vi "lockin_host.vi"() -> ()   [LabVIEW 2009]
uses:
  <vilib>/rvi/interface/nirviOpenFPGA/nirviOpenFPGA.xnode
  FPGA Bitfiles/fpga_lockin.lvproj_FPGA Target_lockin_fpga.vi.lvbitx
  lockin_fpga.vi
  <vilib>/FPGAPlugInAG/Pxi-7841r/nirviIntfOpen_PXI-7841R.vi
  <vilib>/rvi/interface/nirviMethod/nirviMethod.xnode
  <vilib>/Utility/error.llb/Merge Errors.vi
  <vilib>/LabVIEW Targets/FPGA/Rio/nirio_HostInterface/nirio_DMAStopAll.vi
  <vilib>/rvi/interface/common/niFpgaNodeNameForErrorReporting.ctl
  <vilib>/rvi/errors/niLvFpgaWhatHappensToTopLevelVI.ctl
  <vilib>/LabVIEW Targets/FPGA/Rio/nirio_HostInterface/nirio_DisableInterrupts.vi
  <vilib>/Utility/error.llb/Error Cluster From Error Code.vi
  <vilib>/rvi/errors/niLvFpgaAdjustHostInterfaceError.vi
  <vilib>/LabVIEW Targets/FPGA/Rio/nirio_HostInterface/nirio_Reset.vi
  <vilib>/RVI Host/nirviSupport.llb/nirviErrorClusterFromErrorCode.vi
  <vilib>/LabVIEW Targets/FPGA/Rio/nirio_HostInterface/nirio_EnableInterrupts.vi
  <vilib>/rvi/errors/niLvFpgaReportInternalErrorWithAdditionalInfo.vi
  <vilib>/rvi/interface/nirviReadWriteControl/nirviReadWriteControl.xnode
  <vilib>/rvi/interface/nirviCloseFPGA/nirviCloseFPGA.xnode
  <vilib>/FPGAPlugInAG/Pxi-7841r/nirviIntfClose_PXI-7841R.vi
  <vilib>/userDefined/High Color/nirio_resource_hc.ctl
  NiRioSrv.dll
panel:
  in  "Time Constant [s] 4":dbl caption="Time Constant [s]"
  out "Y [V] 4":dbl caption="Y [V]"
  out "Phase [Deg] 4":dbl caption="Phase [Deg]"
  out "R [V] 4":dbl caption="R [V]"
  out "X [V] 4":dbl
  out "Filter Rolloff 4":enum8{"6 dB", "12 dB", "18 dB", "24 dB"}(ring) caption="Filter Rolloff"
  in  "Amplitude [V] 4":dbl caption="Amplitude [V]"
  in  "Frequency [Hz] 4":dbl caption="Frequency [Hz]"
  in  "Phase [Deg] 4":dbl caption="Phase [Deg]"
  in  "Time Constant [s] 3":dbl caption="Time Constant [s]"
  out "Y [V] 3":dbl caption="Y [V]"
  out "Phase [Deg] 3":dbl caption="Phase [Deg]"
  out "R [V] 3":dbl caption="R [V]"
  out "X [V] 3":dbl
  out "Filter Rolloff 3":enum8{"6 dB", "12 dB", "18 dB", "24 dB"}(ring) caption="Filter Rolloff"
  in  "Amplitude [V] 3":dbl caption="Amplitude [V]"
  in  "Frequency [Hz] 3":dbl caption="Frequency [Hz]"
  in  "Phase [Deg] 3":dbl caption="Phase [Deg]"
  in  "Time Constant [s] 2":dbl caption="Time Constant [s]"
  out "Y [V] 2":dbl caption="Y [V]"
  out "Phase [Deg] 2":dbl caption="Phase [Deg]"
  out "R [V] 2":dbl caption="R [V]"
  out "X [V] 2":dbl
  out "Filter Rolloff 2":enum8{"6 dB", "12 dB", "18 dB", "24 dB"}(ring) caption="Filter Rolloff"
  in  "Amplitude [V] 2":dbl caption="Amplitude [V]"
  in  "Frequency [Hz] 2":dbl caption="Frequency [Hz]"
  in  "Phase [Deg] 2":dbl caption="Phase [Deg]"
  in  "Time Constant [s] 1":dbl caption="Time Constant [s]"
  out "Y [V] 1":dbl caption="Y [V]"
  out "Phase [Deg] 1":dbl caption="Phase [Deg]"
  out "R [V] 1":dbl caption="R [V]"
  out "X [V] 1":dbl
  in  "Data Rate [Hz]":dbl
  out "Filter Rolloff 1":enum8{"6 dB", "12 dB", "18 dB", "24 dB"}(ring) caption="Filter Rolloff"
  in  "stop":bool
  in  "Update Freq [Hz]":dbl
  in  "Amplitude [V] 1":dbl caption="Amplitude [V]"
  in  "Frequency [Hz] 1":dbl caption="Frequency [Hz]"
  in  "Phase [Deg] 1":dbl caption="Phase [Deg]"
  # "Lockin Amplifier 1"
  # "Lockin Amplifier 3"
  # "Filter Settings"
  # "Output"
  # "Filter Settings"
  # "Output"
  # "Reference Signal Settings"
  # "Reference Signal Settings"
  # "Lockin Amplifier 2"
  # "Lockin Amplifier 4"
  # "Filter Settings"
  # "Output"
  # "Filter Settings"
  # "Output"
  # "Global"
  # "Reference Signal Settings"
  # "Reference Signal Settings"
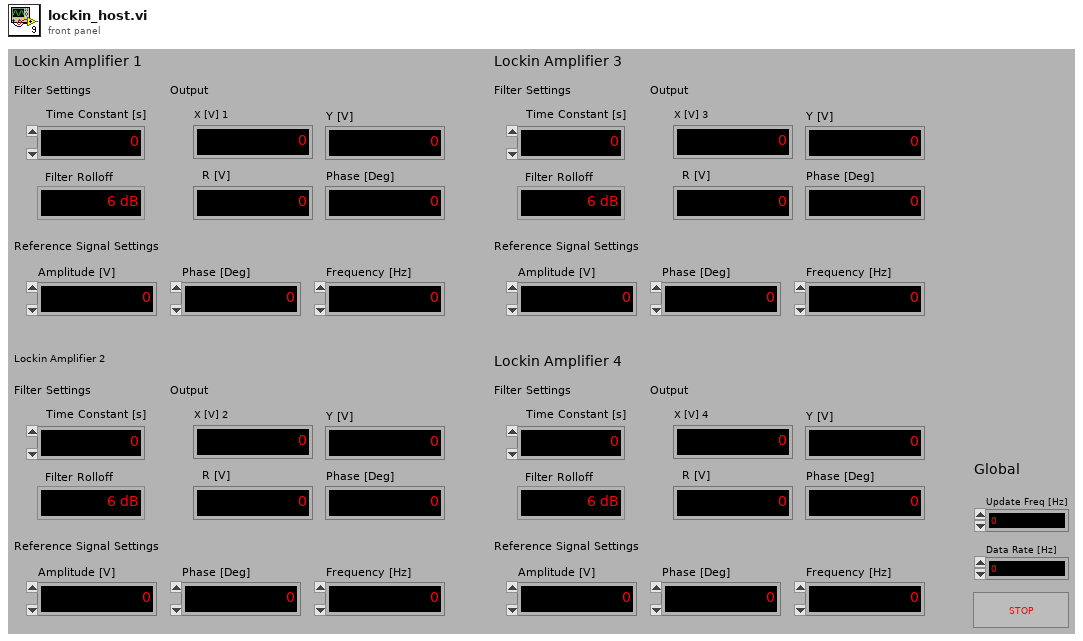
[diagram p1: front panel]
types:
  T1 = typedef "niFpgaNodeNameForErrorReporting.ctl" = enum16{"Open FPGA VI Reference", "Read/Write Control", "Invoke Method: Abort", "Invoke Method: Acknowledge IRQ", "Invoke Method: Download", "Invoke Method: FIFO.Configure", "Invoke Method: FIFO.Read", "Invoke Method: FIFO.Start", "Invoke Method: FIFO.Stop", "Invoke Method: FIFO.Write", "Invoke Method: Reset", "Invoke Method: Run", "Invoke Method: Wait on IRQ", "Close FPGA VI Reference"}
  T2 = typedef "niLvFpgaWhatHappensToTopLevelVI.ctl" = enum16{"top level VI scripted behind XNode", "top level VI inlined behind XNode"}
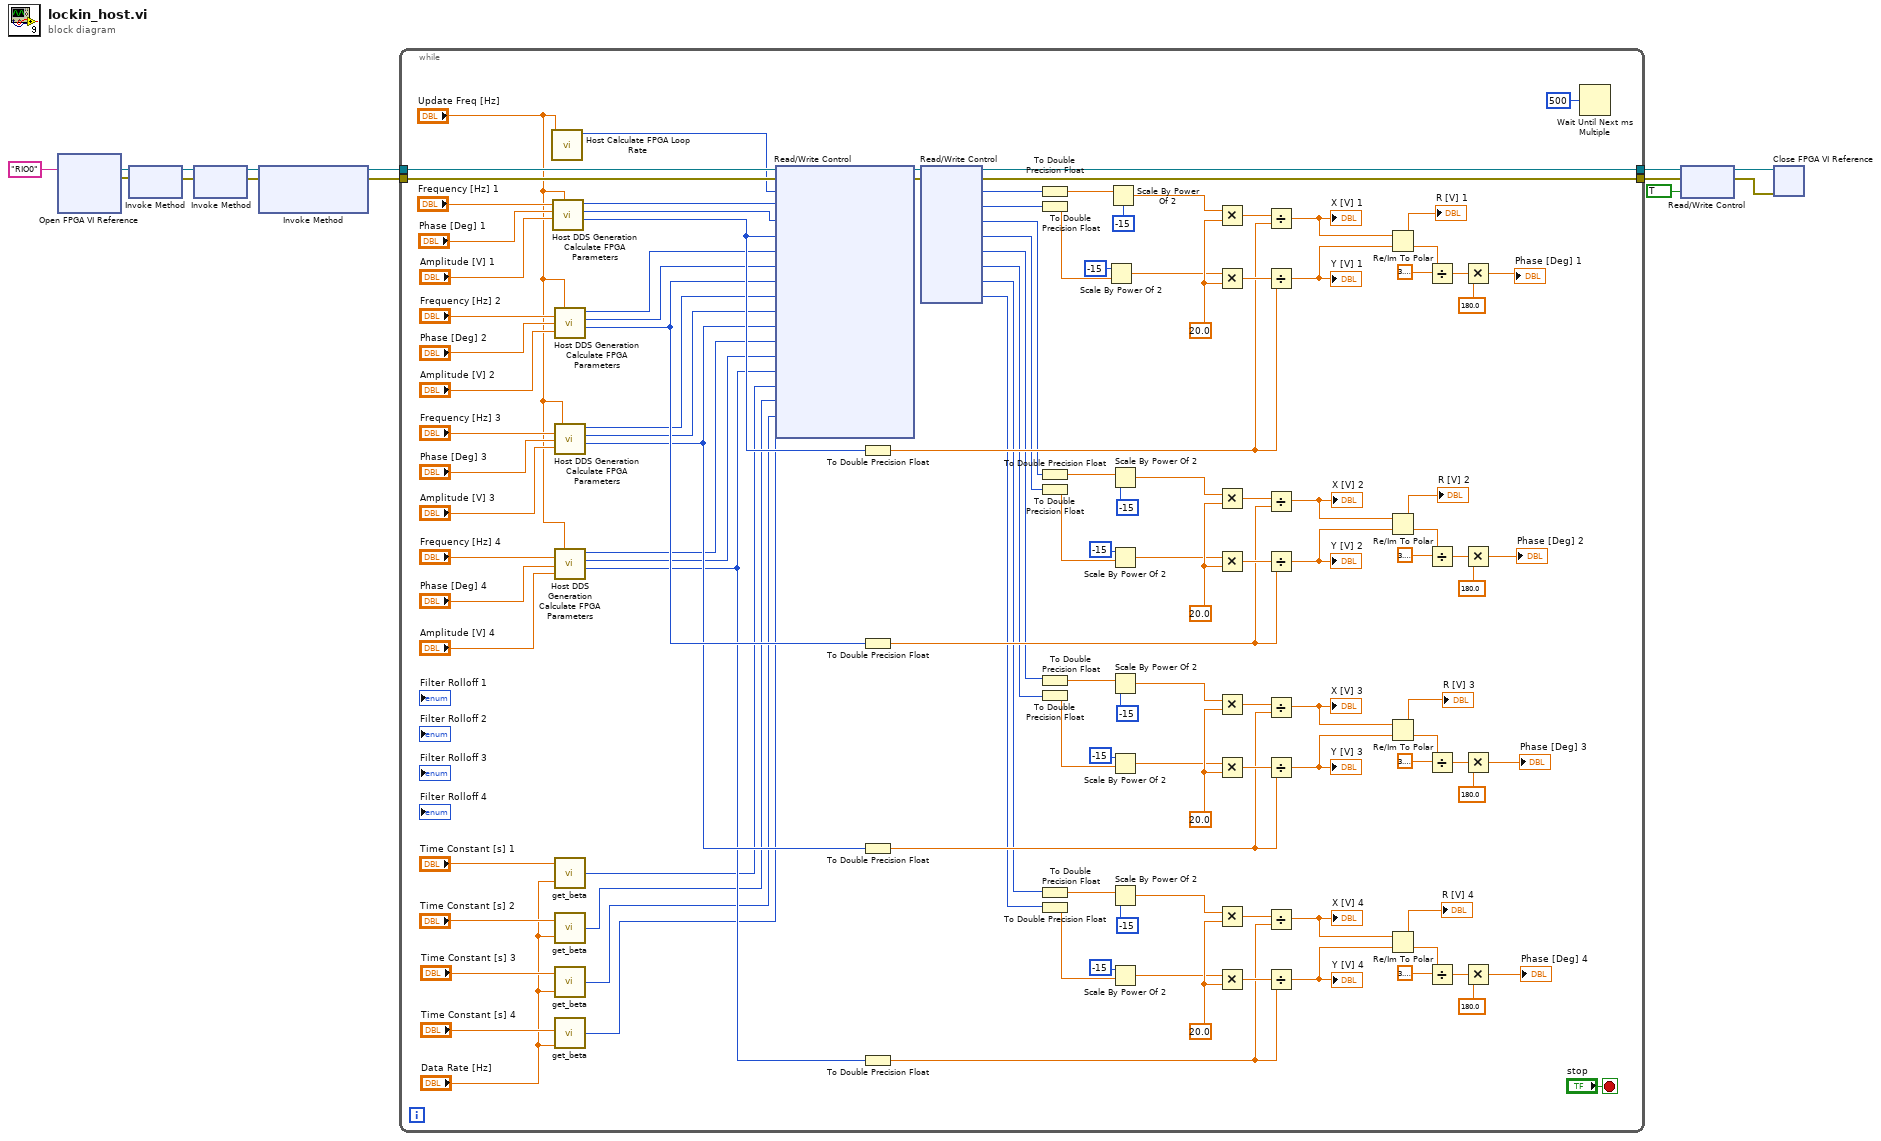
[diagram p0: block diagram]
diagram:
  n1 = xnode "Open FPGA VI Reference"("resource name"="RIO0") -> ("FPGA VI Reference Out"=w9:refnum<k20>, "error out"=w8:errorcluster)  [unwired: 1 in]
  n2 = xnode "Invoke Method"("FPGA VI Reference In"=w9, "error in"=w8) -> ("FPGA VI Reference Out"=w13:refnum<k20>, "error out"=w12:errorcluster)
  n3 = xnode "Invoke Method"("FPGA VI Reference In"=w13, "error in"=w12) -> ("FPGA VI Reference Out"=w11:refnum<k20>, "error out"=w10:errorcluster)
  n4 = xnode "Invoke Method"("FPGA VI Reference In"=w11, "error in"=w10) -> ("FPGA VI Reference Out"=w7:refnum<k20>, "error out"=w6:errorcluster)  [unwired: 1 out]
  n5 = while {
    tunnel: w7 -> [w133]
    tunnel: w6 -> [w132]
    tunnel: [w126] -> w3
    tunnel: [w125] -> w2
    stop <- "stop" stop-if-true
    w44 = 20.0
    w83 = 20.0
    w108 = 20.0
    w100 = 20.0
    n6 = call "Host Calculate FPGA Loop Rate.vi"("Loop Frequency (Hz)"="Update Freq [Hz]") -> ("Loop  Rate (ticks)"=w131:u32)  [unwired: 10 in]
    n7 = call "Host DDS Generation Calculate FPGA Parameters.vi"("Loop Rate (Hz)"="Update Freq [Hz]", "Signal Amplitude (V)"="Amplitude [V] 1", "Phase Shift (Deg)"="Phase [Deg] 1", "DDS Signal Frequency (Hz)"="Frequency [Hz] 1") -> ("AO Amplitude"=w119:u16, "Phase Shift Sin"=w129:u32, "Accumulator Increment"=w130:u32)  [unwired: 3 in, 2 out]
    n8 = call "Host DDS Generation Calculate FPGA Parameters.vi"("Loop Rate (Hz)"="Update Freq [Hz]", "Signal Amplitude (V)"="Amplitude [V] 2", "Phase Shift (Deg)"="Phase [Deg] 2", "DDS Signal Frequency (Hz)"="Frequency [Hz] 2") -> ("AO Amplitude"=w103:u16, "Phase Shift Sin"=w111:u32, "Accumulator Increment"=w112:u32)  [unwired: 3 in, 2 out]
    n9 = call "Host DDS Generation Calculate FPGA Parameters.vi"("Loop Rate (Hz)"="Update Freq [Hz]", "Signal Amplitude (V)"="Amplitude [V] 3", "Phase Shift (Deg)"="Phase [Deg] 3", "DDS Signal Frequency (Hz)"="Frequency [Hz] 3") -> ("AO Amplitude"=w72:u16, "Phase Shift Sin"=w86:u32, "Accumulator Increment"=w87:u32)  [unwired: 3 in, 2 out]
    n10 = call "Host DDS Generation Calculate FPGA Parameters.vi"("Loop Rate (Hz)"="Update Freq [Hz]", "Signal Amplitude (V)"="Amplitude [V] 4", "Phase Shift (Deg)"="Phase [Deg] 4", "DDS Signal Frequency (Hz)"="Frequency [Hz] 4") -> ("AO Amplitude"=w32:u16, "Phase Shift Sin"=w47:u32, "Accumulator Increment"=w48:u32)  [unwired: 3 in, 2 out]
    n11 = call "get_beta.vi"("Data Rate [Hz]"="Data Rate [Hz]", "Time Constant [s]"="Time Constant [s] 1") -> ("beta"=w16:i32)
    n12 = call "get_beta.vi"("Data Rate [Hz]"="Data Rate [Hz]", "Time Constant [s]"="Time Constant [s] 2") -> ("beta"=w17:i32)
    n13 = call "get_beta.vi"("Data Rate [Hz]"="Data Rate [Hz]", "Time Constant [s]"="Time Constant [s] 3") -> ("beta"=w18:i32)
    n14 = call "get_beta.vi"("Data Rate [Hz]"="Data Rate [Hz]", "Time Constant [s]"="Time Constant [s] 4") -> ("beta"=w19:i32)
    n15 = xnode "Read/Write Control"("FPGA VI Reference In"=w133, "error in"=w132, "Update Rate (ticks)"=w131, "Accumulator Increment 1"=w130, "Phase Shift 1"=w129, "Signal Amplitude 1"=w119, "Accumulator Increment 2"=w112, "Phase Shift 2"=w111, "Signal Amplitude 2"=w103, "Accumulator Increment 3"=w87, "Phase Shift 3"=w86, "Signal Amplitude 3"=w72, "Accumulator Increment 4"=w48, "Phase Shift 4"=w47, "Signal Amplitude 4"=w32, "beta1"=w16, "beta2"=w17, "beta3"=w18, "beta4"=w19) -> ("FPGA VI Reference Out"=w128:refnum<k20>, "error out"=w127:errorcluster)
    n16 = To Double Precision Float(number=w119) -> (double precision float=w118:dbl)
    n17 = To Double Precision Float(number=w103) -> (double precision float=w102:dbl)
    n18 = To Double Precision Float(number=w72) -> (double precision float=w71:dbl)
    n19 = To Double Precision Float(number=w32) -> (double precision float=w33:dbl)
    n20 = xnode "Read/Write Control"("FPGA VI Reference In"=w128, "error in"=w127) -> ("FPGA VI Reference Out"=w126:refnum<k20>, "error out"=w125:errorcluster, "X_fpga 1"=w27:i32, "Y_fpga 1"=w26:i32, "X_fpga 2"=w25:i32, "Y_fpga 2"=w24:i32, "X_fpga 3"=w23:i32, "Y_fpga 3"=w22:i32, "X_fpga 4"=w21:i32, "Y_fpga 4"=w20:i32)
    n21 = To Double Precision Float(number=w27) -> (double precision float=w96:dbl)
    n22 = To Double Precision Float(number=w26) -> (double precision float=w98:dbl)
    n23 = To Double Precision Float(number=w25) -> (double precision float=w93:dbl)
    n24 = To Double Precision Float(number=w24) -> (double precision float=w90:dbl)
    n25 = To Double Precision Float(number=w23) -> (double precision float=w78:dbl)
    n26 = To Double Precision Float(number=w22) -> (double precision float=w75:dbl)
    n27 = To Double Precision Float(number=w21) -> (double precision float=w39:dbl)
    n28 = To Double Precision Float(number=w20) -> (double precision float=w36:dbl)
    n29 = Scale By Power Of 2(n=-15, x=w98) -> (x*2^n=w99:dbl)
    n30 = Scale By Power Of 2(n=-15, x=w96) -> (x*2^n=w94:dbl)
    n31 = Scale By Power Of 2(n=-15, x=w93) -> (x*2^n=w92:dbl)
    n32 = Scale By Power Of 2(n=-15, x=w90) -> (x*2^n=w89:dbl)
    n33 = Scale By Power Of 2(n=-15, x=w78) -> (x*2^n=w77:dbl)
    n34 = Scale By Power Of 2(n=-15, x=w75) -> (x*2^n=w74:dbl)
    n35 = Scale By Power Of 2(n=-15, x=w39) -> (x*2^n=w38:dbl)
    n36 = Scale By Power Of 2(n=-15, x=w36) -> (x*2^n=w35:dbl)
    n37 = Multiply(x=w94, y=w100) -> (x*y=w124:dbl)
    n38 = Multiply(x=w99, y=w100) -> (x*y=w123:dbl)
    n39 = Multiply(x=w92, y=w108) -> (x*y=w110:dbl)
    n40 = Multiply(x=w89, y=w108) -> (x*y=w109:dbl)
    n41 = Multiply(x=w77, y=w83) -> (x*y=w85:dbl)
    n42 = Multiply(x=w74, y=w83) -> (x*y=w84:dbl)
    n43 = Multiply(x=w38, y=w44) -> (x*y=w46:dbl)
    n44 = Multiply(x=w35, y=w44) -> (x*y=w45:dbl)
    n45 = Divide(x=w124, y=w118) -> (x/y=w122:dbl)
    "X [V] 1" <- w122
    n46 = Divide(x=w123, y=w118) -> (x/y=w121:dbl)
    "Y [V] 1" <- w121
    n47 = Divide(x=w110, y=w102) -> (x/y=w54:dbl)
    "X [V] 2" <- w54
    n48 = Divide(x=w109, y=w102) -> (x/y=w55:dbl)
    "Y [V] 2" <- w55
    n49 = Divide(x=w85, y=w71) -> (x/y=w61:dbl)
    "X [V] 3" <- w61
    n50 = Divide(x=w84, y=w71) -> (x/y=w60:dbl)
    "Y [V] 3" <- w60
    n51 = Divide(x=w46, y=w33) -> (x/y=w31:dbl)
    "X [V] 4" <- w31
    n52 = Divide(x=w45, y=w33) -> (x/y=w30:dbl)
    "Y [V] 4" <- w30
    n53 = Re/Im To Polar(2:w121, 3:w122) -> (0:w117:dbl, 1:→"R [V] 1":dbl)
    n54 = Re/Im To Polar(2:w55, 3:w54) -> (0:w107:dbl, 1:→"R [V] 2":dbl)
    n55 = Re/Im To Polar(2:w60, 3:w61) -> (0:w82:dbl, 1:→"R [V] 3":dbl)
    n56 = Re/Im To Polar(2:w30, 3:w31) -> (0:w43:dbl, 1:→"R [V] 4":dbl)
    n57 = Divide(x=w117, y=3.141592653589793) -> (x/y=w115:dbl)
    n58 = Divide(x=w107, y=3.141592653589793) -> (x/y=w105:dbl)
    n59 = Divide(x=w82, y=3.141592653589793) -> (x/y=w80:dbl)
    n60 = Divide(x=w43, y=3.141592653589793) -> (x/y=w41:dbl)
    n61 = Multiply(x=w115, y=180.0) -> (x*y=→"Phase [Deg] 1":dbl)
    n62 = Multiply(x=w105, y=180.0) -> (x*y=→"Phase [Deg] 2":dbl)
    n63 = Multiply(x=w80, y=180.0) -> (x*y=→"Phase [Deg] 3":dbl)
    n64 = Multiply(x=w41, y=180.0) -> (x*y=→"Phase [Deg] 4":dbl)
    n65 = Wait Until Next ms Multiple(millisecond multiple=u32 500) -> ()  [unwired: 1 out]
  }
  n66 = xnode "Read/Write Control"("FPGA VI Reference In"=w3, "error in"=w2, "stop"=TRUE) -> ("FPGA VI Reference Out"=w5:refnum<k20>, "error out"=w4:errorcluster)
  n67 = xnode "Close FPGA VI Reference"("FPGA VI Reference In"=w5, "error in"=w4) -> ()  [unwired: 1 out]
